vi "SPI MPU9250.vi"() -> ()   [LabVIEW 2023, in "CTI-Visa-Scratchpad.lvlib"]
uses:
  CTI-Visa-Scratchpad.lvlib
  CTI-Visa/SPI Config.ctl
  6879a345-385a-4bff-b9a2-dde094eab613.vi
  CTI-Visa/CTI-Visa.lvlib
  CTI-Visa-DeviceLib/CTI-Visa-DeviceLib.lvlib
panel:
  out "ID":string
  out "Chart":T1(graph)
  in  "stop":bool
  out "error out":errorcluster={"status"=TRUE, "code"=-1073807339, "source"="VISA Read in CTI-Visa.lvlib:Read Block.vi->CTI-Visa.lvlib:Read SPI.vi->CTI-Visa-DeviceLib.lvlib:SPI Read Register.vi->CTI-Visa-Scratchpad.lvlib:SPI MPU9250.vi"}
  in  "CS Pin":i32=5
  in  "Baud":u32=500000 format="%.0p"
  in  "Bus":u8
  in  "SPI Config":T2={"Mode"=0, "Data Bits"=8, "MOSI Pin"=7, "MISO Pin"=4, "SCK Pin"=6}
  in  "Port":refnum<visa-resource-name>="COM4"
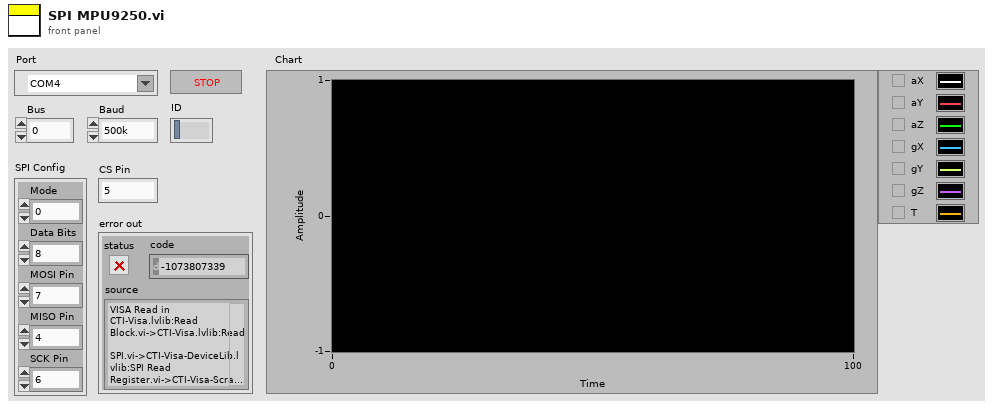
[diagram p1: front panel]
types:
  T1 = cluster{"X":u16, "Y":u16, "Z":u16, "X":u16, "Y":u16, "Z":u16, "T":u16}
  T2 = typedef "CTI-Visa.lvlib/SPI Config.ctl" = cluster{"Mode":u8, "Data Bits":u8, "MOSI Pin":u8, "MISO Pin":u8, "SCK Pin":u8}
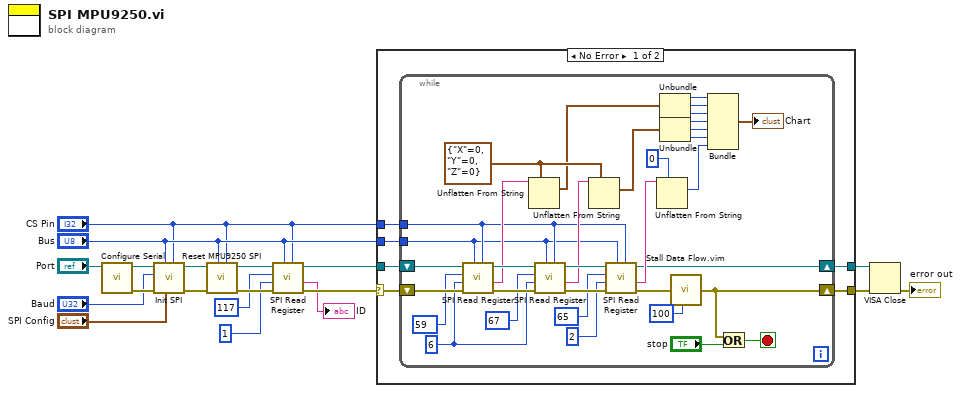
[diagram p0: block diagram]
diagram:
  n1 = call "Configure Serial.vi"("VISA resource name in"="Port") -> ("error out"=w18:errorcluster, "VISA resource name"=w17:refnum<visa-resource-name>)  [unwired: 9 in]
  n2 = call "Init SPI.vi"("CS GPIO (None)"="CS Pin", "SPI Config"="SPI Config", "Bus"="Bus", "error in (no error)"=w18, "Baud"="Baud", "VISA resource name in"=w17) -> ("error out"=w3:errorcluster, "VISA resource name"=w4:refnum<visa-resource-name>)  [unwired: 4 in]
  n3 = call "Reset MPU9250 SPI.vi"("CS Pin"="CS Pin", "Bus"="Bus", "error in (no error)"=w3, "VISA resource name in"=w4) -> ("error out"=w13:errorcluster, "VISA resource name"=w11:refnum<visa-resource-name>)  [unwired: 6 in]
  n4 = call "SPI Read Register.vi"("CS GPIO (None)"="CS Pin", "Bus"="Bus", "error in (no error)"=w13, "Len"=u8 1, "Register"=u8 117, "VISA resource name in"=w11) -> ("error out"=w12:errorcluster, "Data"=→"ID":string, "VISA resource name"=w10:refnum<visa-resource-name>)  [unwired: 3 in]
  n5 = case shown="No Error" w12 {
    selector: w12 -> [w25 w60]
    tunnel: w10 -> [w24 w61]
    tunnel: [w23 w61] -> w16
    tunnel: [w22 w60] -> w15
    tunnel: "CS Pin" -> [w21 _]
    tunnel: "Bus" -> [w20 _]
    frame No Error {
      n6 = while {
        shift-right: [w50] -> w22
        shift-left: w25 -> [w59]
        shift-right: [w32] -> w23
        shift-left: w24 -> [w34]
        tunnel: w21 -> [w30]
        tunnel: w20 -> [w29]
        stop <- w51 stop-if-true
        w46 = cluster{"X":u16, "Y":u16, "Z":u16} {"X"=0, "Y"=0, "Z"=0}
        w55 = u8 6 ("Len")
        n7 = call "SPI Read Register.vi"("CS GPIO (None)"=w30, "Bus"=w29, "error in (no error)"=w59, "Len"=w55, "Register"=u8 59, "VISA resource name in"=w34) -> ("error out"=w56:errorcluster, "Data"=w48:string, "VISA resource name"=w57:refnum<visa-resource-name>)  [unwired: 3 in]
        n8 = Unflatten From String(type=w46, binary string=w48) -> (value=w43:cluster{"X":u16, "Y":u16, "Z":u16})  [unwired: 3 in, 2 out]
        n9 = call "SPI Read Register.vi"("CS GPIO (None)"=w30, "Bus"=w29, "error in (no error)"=w56, "Len"=w55, "Register"=u8 67, "VISA resource name in"=w57) -> ("error out"=w53:errorcluster, "Data"=w47:string, "VISA resource name"=w54:refnum<visa-resource-name>)  [unwired: 3 in]
        n10 = Unflatten From String(type=w46, binary string=w47) -> (value=w42:cluster{"X":u16, "Y":u16, "Z":u16})  [unwired: 3 in, 2 out]
        n11 = call "SPI Read Register.vi"("CS GPIO (None)"=w30, "Bus"=w29, "error in (no error)"=w53, "Len"=u8 2, "Register"=u8 65, "VISA resource name in"=w54) -> ("error out"=w33:errorcluster, "Data"=w44:string, "VISA resource name"=w32:refnum<visa-resource-name>)  [unwired: 3 in]
        n12 = Unflatten From String(type=u16 0 ("T"), binary string=w44) -> (value=w35:u16)  [unwired: 3 in, 2 out]
        n13 = Unbundle(w43) -> ("X"=w41:u16, "Y"=w40:u16, "Z"=w39:u16)
        n14 = Unbundle(w42) -> ("X"=w38:u16, "Y"=w37:u16, "Z"=w36:u16)
        n15 = call "Stall Data Flow.vim"("value in"=w33, "milliseconds to wait"=u32 100) -> ("value out"=w50:errorcluster)  [unwired: 1 out]
        n16 = Bundle("X"=w41, "Y"=w40, "Z"=w39, "X"=w38, "Y"=w37, "Z"=w36, "T"=w35) -> (→"Chart":T1)  [unwired: 1 in]
        n17 = Or(x=w50, y="stop") -> (x .or. y?=w51:bool)
      }
    }
    frame Error {
    }
  }
  n18 = VISA Close(VISA resource name=w16, error in (no error)=w15) -> (error out=→"error out":errorcluster)
